vi "1.3.14-ReadWrite.vi"(0 "Read FIFO":refnum<k21>="2.3.2-Lidar Read", 1 "baud rate (9600) 2":u32=9600, 2 "data bits (8) 2":i32=8 min=5 max=8 step=1, 3 "stop bits (10: 1 bit) 2":u16(ring)=10 items=["1.0"=10, "1.5"=15, "2.0"=20], 5 "Write FIFO":refnum<k21>="2.3.1-Lidar Write", 7 "Rx FPGA I/O":refnum<k21>="Rx", 9 "Tx FPGA I/O":refnum<k21>="Tx", 11 "stop bits (10: 1 bit)":u16(ring)=10 items=["1.0"=10, "1.5"=15, "2.0"=20], 12 "Invert Polarity?":bool, 13 "parity (0:none)":enum16{"None", "Odd", "Even", "Mark", "Space"}(ring), 14 "Invert Polarity? 2":bool) -> (4 "Read: Transmission Error":bool, 6 "Read: Transmission Error 2":bool)   [LabVIEW 2010]
uses:
  <vilib>/eio/EIONode/EIONode.xnode
  <vilib>/rvi/eio/nirviEIOImplementation/nirviEIOImplementation.xnode
  <vilib>/rvi/eio/common/nirviEmuClasses.ctl
  <vilib>/rvi/DataTransferAndStorage/Container/XNode/niFpgaContainer.xnode
  <vilib>/rvi/DataTransferAndStorage/Container/Common/niFpgaTransferTypeControl.ctl
  <vilib>/rvi/FIFO/Fifo_Types/niFpgaFifoControlLogicControl.ctl
  <vilib>/rvi/DataTransferAndStorage/Container/Common/niFpgaContainerMethod.ctl
  <vilib>/rvi/DataTransferAndStorage/Container/Common/niFpgaContainerMetaDataKey.ctl
  <vilib>/rvi/DataTransferAndStorage/FIFO/niFpgaPeerToPeerStreamState.ctl
  1.0-Hindbrain Global.vi
  <vilib>/rvi/eio/common/nirviEmuTemplateMethod_noerrors.vi
  <vilib>/rvi/DataTransferAndStorage/Container/Common/niFpgaContainerExecOnDevCompGetState.vi
  <vilib>/rvi/FIFO/Fifo_Resource/nirvififoEmulationSetSize.vi
  <vilib>/rvi/DataTransferAndStorage/Container/Common/niFpgaContainerGetUniqueNameForEmu.vi
  <vilib>/rvi/interface/RandomDataEmulation/nirviRandomDataFPGAFIFO.vi
  <vilib>/rvi/interface/RandomDataEmulation/niFpgaRandomDataHandleErrors.vi
  <vilib>/rvi/eio/common/nirviEmuReportErrorAndStop.vi
panel:
  in  "parity (0:none) 2":enum16{"None", "Odd", "Even", "Mark", "Space"}(ring)
  in  "data bits (8)":i32=8 min=5 max=8 step=1
  in  "baud rate (9600)":u32=9600
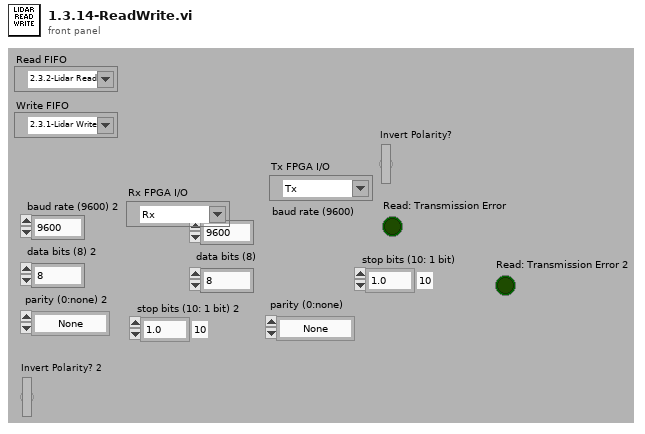
[diagram p1: front panel]
types:
  T1 = typedef "nirviEmuClasses.ctl" = enum16{"IO Read", "IO Write", "Method", "Property Read", "Property Write"}
  T2 = typedef "niFpgaFifoControlLogicControl.ctl" = enum16{"Slice Fabric", "Target Optimal", "Built-in"}
  T3 = typedef "niFpgaContainerMethod.ctl" = enum16{"<none>", "write", "read", "clear", "getNumberOfElementsToWrite", "getNumberOfElementsToRead", "enable", "disable", "flushAndDisable", "getStreamState", "readA", "readB", "dramWrite", "dramWriteWithByteEnables", "dramRequestData", "dramRetrieveData"}
  T4 = typedef "niFpgaTransferTypeControl.ctl" = enum16{"Target-Scoped", "Host to Target - DMA", "Target to Host - DMA", "Peer to Peer Reader", "Peer to Peer Writer", "Bidirectional"}
  T5 = typedef "niFpgaPeerToPeerStreamState.ctl" = enum16{"Unlinked", "Disabled", "Enabled", "Flushing"}
  T6 = typedef "niFpgaContainerMetaDataKey.ctl" = enum16{"FPGA FIFO", "FPGA Memory", "FPGA Register"}
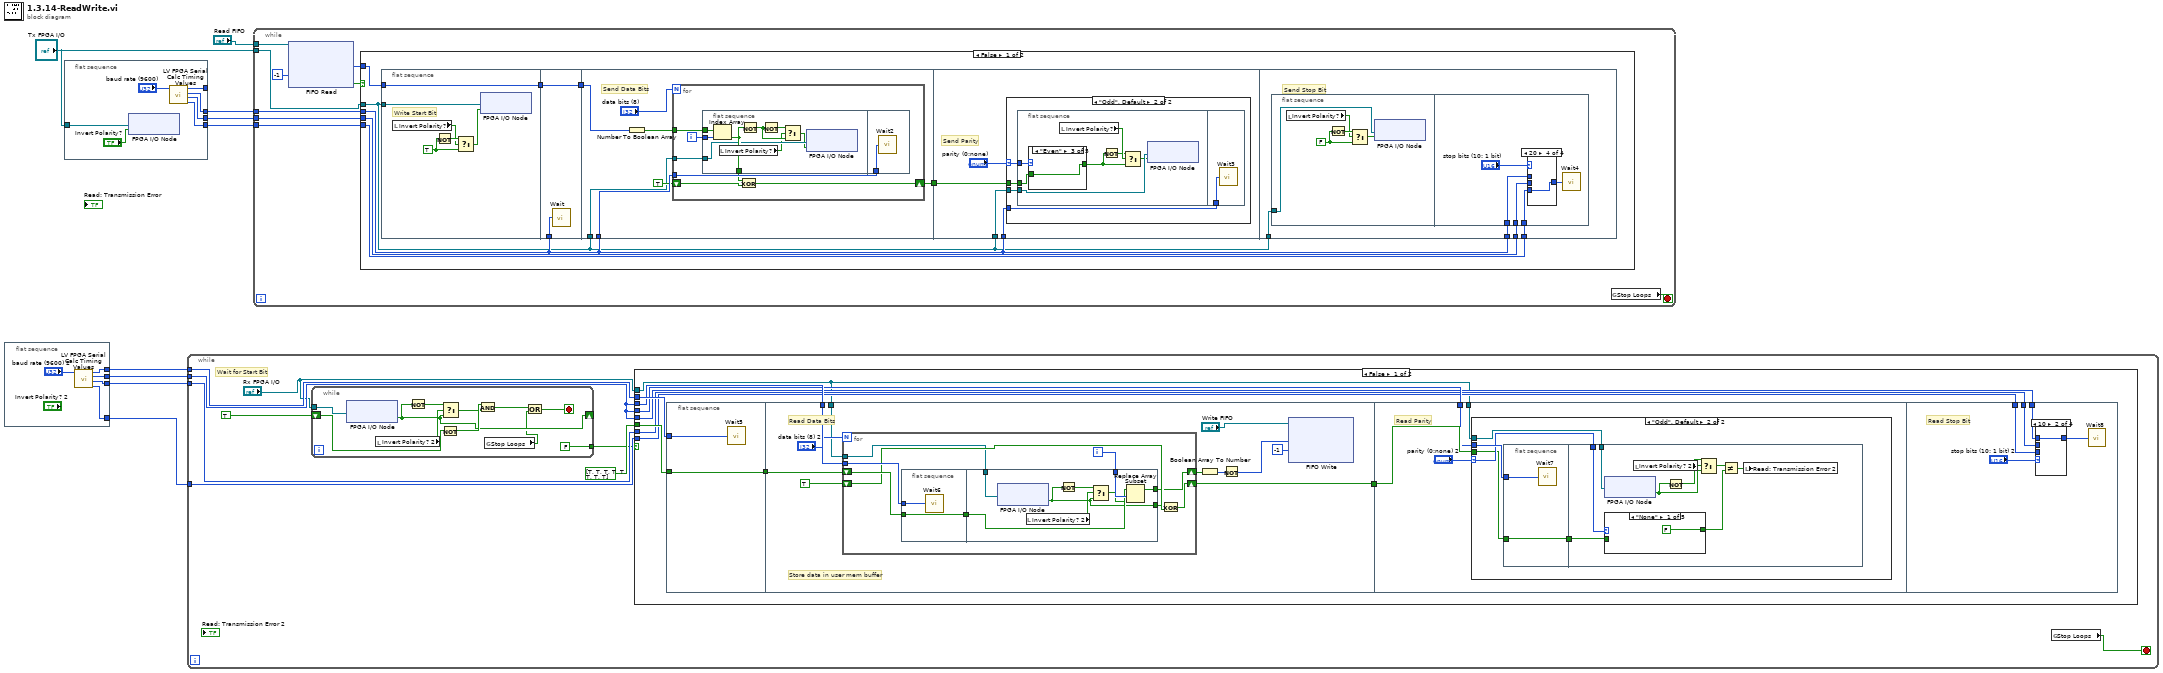
[diagram p0: block diagram]
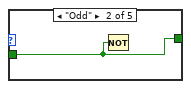
[diagram p3: hidden frame]
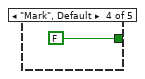
[diagram p5: hidden frame]
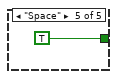
[diagram p6: hidden frame]
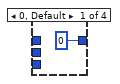
[diagram p7: hidden frame]
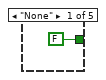
[diagram p12: hidden frame]
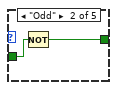
[diagram p13: hidden frame]
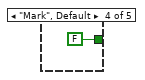
[diagram p14: hidden frame]
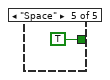
[diagram p15: hidden frame]
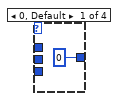
[diagram p16: hidden frame]
diagram:
  n1 = flat-sequence {
    tunnel: [w10] -> w3
    tunnel: [w13] -> w2
    tunnel: [w12] -> w4
    tunnel: [w11] -> w5
    frame #0 {
      n2 = call "LV FPGA Serial Calc Timing Values.vi"("baud rate (1000000)"="baud rate (9600) 2") -> ("Two Bit"=w11:u32, "One and Half Bit"=w12:u32, "One Bit"=w10:u32, "Half Bit"=w13:u32)  [unwired: 1 in, 2 out]
    }
  }
  n3 = flat-sequence {
    tunnel: [w17] -> w9
    tunnel: [w20] -> _
    tunnel: [w19] -> w8
    tunnel: [w18] -> w7
    tunnel: "Tx FPGA I/O" -> [w16]
    frame #0 {
      n4 = xnode "FPGA I/O Node"("I/O Item"="Invert Polarity?", "FPGA I/O In"=w16) -> ()  [unwired: 1 out]
      n5 = call "LV FPGA Serial Calc Timing Values.vi"("baud rate (1000000)"="baud rate (9600)") -> ("Two Bit"=w18:u32, "One and Half Bit"=w19:u32, "One Bit"=w17:u32, "Half Bit"=w20:u32)  [unwired: 1 in, 2 out]
    }
  }
  n6 = while {
    tunnel: w5 -> [w40]
    tunnel: w4 -> [w39]
    tunnel: w3 -> [w38]
    tunnel: w2 -> [w37]
    stop <- w34 stop-if-true
    # "Wait for Start Bit"
    n7 = while {
      tunnel: [FALSE] -> w36
      shift-right: [w43] -> _
      shift-left: TRUE -> [w51]
      tunnel: "Rx FPGA I/O" -> [w47]
      stop <- w48 stop-if-true
      n8 = xnode "FPGA I/O Node"("FPGA I/O In"=w47) -> ("I/O Item"=w43:bool)  [unwired: 1 out]
      n9 = local read "Invert Polarity? 2"() -> (w45:bool)
      n10 = Not(x=w43) -> (.not. x?=w46:bool)
      n11 = Not(x=w51) -> (.not. x?=w50:bool)
      n12 = Select(t=w46, s=w45, f=w43) -> (s? t:f=w44:bool)
      n13 = And(x=w50, y=w44) -> (x .and. y?=w49:bool)
      n14 = global read "1.0-Hindbrain Global.vi" "Stop Loops"() -> (w42:bool)
      n15 = Or(x=w49, y=w42) -> (x .or. y?=w48:bool)
    }
    n16 = case shown="False" w36 {
      tunnel: bool[] [TRUE, TRUE, TRUE, TRUE, TRUE, TRUE, TRUE, TRUE] -> [w80 _]
      tunnel: w37 -> [w79 _]
      tunnel: w38 -> [w78 _]
      tunnel: w38 -> [w77 _]
      tunnel: w38 -> [w76 _]
      tunnel: w39 -> [w75 _]
      tunnel: w40 -> [w74 _]
      tunnel: "Rx FPGA I/O" -> [w72 _]
      frame False {
        n17 = flat-sequence {
          tunnel: [w83] -> w81
          tunnel: w80 -> [w83]
          tunnel: w79 -> [w82]
          tunnel: w81 -> [w94]
          tunnel: w78 -> [w93]
          tunnel: [w89] -> w73
          tunnel: w72 -> [w87]
          tunnel: w77 -> [w451]
          tunnel: w73 -> [w453]
          tunnel: w72 -> [w450]
          tunnel: w76 -> [w497]
          tunnel: w75 -> [w496]
          tunnel: w74 -> [w495]
          frame #0 {
            n18 = call "Wait5"("Count(Ticks)"=w82) -> ()  [unwired: 1 out]
          }
          frame #1 {
            # "Store data in user mem buffer"
            # "Read Data Bits"
            n19 = for {
              N: "data bits (8) 2" -> [_]
              shift-right: [w414] -> w92
              shift-left: w94 -> [w420]
              tunnel: w93 -> [w418]
              shift-right: [w417] -> w89
              shift-left: TRUE -> [w416]
              tunnel: w87 -> [w412]
              i -> [w413]
              n20 = flat-sequence {
                tunnel: w420 -> [w422]
                tunnel: [w422] -> w419
                tunnel: w418 -> [w421]
                tunnel: w413 -> [w430]
                tunnel: w419 -> [w429]
                tunnel: [w428] -> w414
                tunnel: [w423] -> w415
                tunnel: w412 -> [w427]
                frame #0 {
                  n21 = call "Wait6"("Count(Ticks)"=w421) -> ()  [unwired: 1 out]
                }
                frame #1 {
                  n22 = xnode "FPGA I/O Node"("FPGA I/O In"=w427) -> ("I/O Item"=w423:bool)  [unwired: 1 out]
                  n23 = local read "Invert Polarity? 2"() -> (w426:bool)
                  n24 = Not(x=w423) -> (.not. x?=w425:bool)
                  n25 = Select(t=w425, s=w426, f=w423) -> (s? t:f=w424:bool)
                  n26 = Replace Array Subset(array=w429, new element=w424, index=w430) -> (w428:bool[])
                }
              }
              n27 = Exclusive Or(1:w416, 2:w415) -> (0:w417:bool)
            }
            n28 = Boolean Array To Number(Boolean array=w92) -> (number=w91:u8)
            n29 = Not(x=w91) -> (.not. x?=w86:u8)
            n30 = xnode ("FIFO Write")("Element"=w86, "Timeout"=-1, "FIFO In"="Write FIFO") -> ()  [unwired: 2 out]
          }
          frame #2 {
            # "Read Parity"
            n31 = case shown="\"Odd\", Default" "parity (0:none) 2" {
              selector: "parity (0:none) 2" -> [_ w457]
              tunnel: w453 -> [_ w455]
              tunnel: w451 -> [_ w458]
              tunnel: w450 -> [_ w454]
              frame "None" {
              }
              frame "Odd", Default {
                n32 = flat-sequence {
                  tunnel: w458 -> [w460]
                  tunnel: [w459] -> w456
                  tunnel: w455 -> [w459]
                  tunnel: w457 -> [w469]
                  tunnel: w456 -> [w467]
                  tunnel: w454 -> [w465]
                  frame #0 {
                    n33 = call "Wait7"("Count(Ticks)"=w460) -> ()  [unwired: 1 out]
                  }
                  frame #1 {
                    n34 = xnode "FPGA I/O Node"("FPGA I/O In"=w465) -> ("I/O Item"=w462:bool)  [unwired: 1 out]
                    n35 = case shown="\"None\"" w469 {
                      tunnel: w467 -> [_ w490 w491 _ _]
                      tunnel: [FALSE ("y") w490 w491 FALSE ("y") TRUE ("y")] -> w468
                      frame "None" {
                      }
                      frame "Odd" {
                        n36 = Not(x=w490) -> ()  [unwired: 1 out]
                      }
                      frame "Even" {
                      }
                      frame "Mark", Default {
                      }
                      frame "Space" {
                      }
                    }
                    n37 = local read "Invert Polarity? 2"() -> (w463:bool)
                    n38 = Not(x=w462) -> (.not. x?=w464:bool)
                    n39 = Select(t=w464, s=w463, f=w462) -> (s? t:f=w461:bool)
                    n40 = Not Equal?(x=w461, y=w468) -> (x != y?=w466:bool)
                    n41 = local write "Read: Transmission Error 2"(w466) -> ()
                  }
                }
              }
            }
          }
          frame #3 {
            # "Read Stop Bit"
            n42 = case shown="10" "stop bits (10: 1 bit) 2" {
              tunnel: w497 -> [_ w500 _ _]
              tunnel: w496 -> [_ _ w501 _]
              tunnel: w495 -> [_ _ _ w502]
              tunnel: [u32 0 ("One Bit") w500 w501 w502] -> w494
              frame 0, Default {
              }
              frame 10 {
              }
              frame 15 {
              }
              frame 20 {
              }
            }
            n43 = call "Wait8"("Count(Ticks)"=w494) -> ()  [unwired: 1 out]
          }
        }
      }
      frame True {
      }
    }
    n44 = global read "1.0-Hindbrain Global.vi" "Stop Loops"() -> (w34:bool)
  }
  n45 = while {
    tunnel: w7 -> [w511]
    tunnel: w8 -> [w510]
    tunnel: w9 -> [w509]
    tunnel: "Tx FPGA I/O" -> [w508]
    tunnel: "Read FIFO" -> [w503]
    stop <- w504 stop-if-true
    n46 = xnode ("FIFO Read")("Timeout"=-1, "FIFO In"=w503) -> ("Element"=w507:u8, "Timed Out?"=w505:bool)  [unwired: 1 out]
    n47 = case shown="False" w505 {
      tunnel: w511 -> [w833 _]
      tunnel: w510 -> [w832 _]
      tunnel: w509 -> [w831 _]
      tunnel: w508 -> [w830 _]
      tunnel: w507 -> [w829 _]
      frame False {
        n48 = flat-sequence {
          tunnel: w830 -> [w842]
          tunnel: w829 -> [w837]
          tunnel: [w837] -> w836
          tunnel: w831 -> [w855]
          tunnel: [w854] -> w835
          tunnel: w836 -> [w854]
          tunnel: w831 -> [w862]
          tunnel: [w860] -> w834
          tunnel: w830 -> [w858]
          tunnel: w835 -> [w857]
          tunnel: w831 -> [w892]
          tunnel: w834 -> [w893]
          tunnel: w830 -> [w891]
          tunnel: w831 -> [w926]
          tunnel: w832 -> [w925]
          tunnel: w833 -> [w924]
          tunnel: w830 -> [w923]
          frame #0 {
            w840 = TRUE
            # "Write Start Bit"
            n49 = local read "Invert Polarity?"() -> (w839:bool)
            n50 = Not(x=w840) -> (.not. x?=w841:bool)
            n51 = Select(t=w841, s=w839, f=w840) -> (s? t:f=w838:bool)
            n52 = xnode "FPGA I/O Node"("I/O Item"=w838, "FPGA I/O In"=w842) -> ()  [unwired: 1 out]
          }
          frame #1 {
            n53 = call "Wait"("Count(Ticks)"=w855) -> ()  [unwired: 1 out]
          }
          frame #2 {
            # "Send Data Bits"
            n54 = Number To Boolean Array(number=w857) -> (Boolean array=w859:bool[])
            n55 = for {
              N: "data bits (8)" -> [_]
              tunnel: w862 -> [w866]
              shift-right: [w869] -> w860
              shift-left: TRUE -> [w868]
              tunnel: w859 -> [w865]
              tunnel: w858 -> [w863]
              i -> [w867]
              n56 = flat-sequence {
                tunnel: w867 -> [w877]
                tunnel: w865 -> [w876]
                tunnel: [w875] -> w864
                tunnel: w863 -> [w874]
                tunnel: w866 -> [w889]
                frame #0 {
                  n57 = Index Array(array=w876, index=w877) -> (element=w875:bool)
                  n58 = local read "Invert Polarity?"() -> (w871:bool)
                  n59 = Not(x=w875) -> (.not. x?=w872:bool)
                  n60 = Not(x=w872) -> (.not. x?=w873:bool)
                  n61 = Select(t=w873, s=w871, f=w872) -> (s? t:f=w870:bool)
                  n62 = xnode "FPGA I/O Node"("I/O Item"=w870, "FPGA I/O In"=w874) -> ()  [unwired: 1 out]
                }
                frame #1 {
                  n63 = call "Wait2"("Count(Ticks)"=w889) -> ()  [unwired: 1 out]
                }
              }
              n64 = Exclusive Or(1:w868, 2:w864) -> (0:w869:bool)
            }
          }
          frame #3 {
            # "Send Parity"
            n65 = case shown="\"Odd\", Default" "parity (0:none)" {
              selector: "parity (0:none)" -> [_ w897]
              tunnel: w893 -> [_ w896]
              tunnel: w892 -> [_ w895]
              tunnel: w891 -> [_ w894]
              frame "None" {
              }
              frame "Odd", Default {
                n66 = flat-sequence {
                  tunnel: w896 -> [w903]
                  tunnel: w897 -> [w904]
                  tunnel: w894 -> [w902]
                  tunnel: w895 -> [w922]
                  frame #0 {
                    n67 = case shown="\"Even\"" w904 {
                      tunnel: w903 -> [_ w918 w919 _ _]
                      tunnel: [FALSE ("y") w917 w919 FALSE ("y") TRUE ("y")] -> w899
                      frame "None" {
                      }
                      frame "Odd" {
                        n68 = Not(x=w918) -> (.not. x?=w917:bool)
                      }
                      frame "Even" {
                      }
                      frame "Mark", Default {
                      }
                      frame "Space" {
                      }
                    }
                    n69 = local read "Invert Polarity?"() -> (w901:bool)
                    n70 = Not(x=w899) -> (.not. x?=w900:bool)
                    n71 = Select(t=w900, s=w901, f=w899) -> (s? t:f=w898:bool)
                    n72 = xnode "FPGA I/O Node"("I/O Item"=w898, "FPGA I/O In"=w902) -> ()  [unwired: 1 out]
                  }
                  frame #1 {
                    n73 = call "Wait3"("Count(Ticks)"=w922) -> ()  [unwired: 1 out]
                  }
                }
              }
            }
          }
          frame #4 {
            # "Send Stop Bit"
            n74 = flat-sequence {
              tunnel: w923 -> [w931]
              tunnel: w926 -> [w947]
              tunnel: w925 -> [w946]
              tunnel: w924 -> [w945]
              frame #0 {
                w929 = FALSE
                n75 = local read "Invert Polarity?"() -> (w928:bool)
                n76 = Not(x=w929) -> (.not. x?=w930:bool)
                n77 = Select(t=w930, s=w928, f=w929) -> (s? t:f=w927:bool)
                n78 = xnode "FPGA I/O Node"("I/O Item"=w927, "FPGA I/O In"=w931) -> ()  [unwired: 1 out]
              }
              frame #1 {
                n79 = case shown="20" "stop bits (10: 1 bit)" {
                  tunnel: w947 -> [_ w949 _ _]
                  tunnel: w946 -> [_ _ w950 _]
                  tunnel: w945 -> [_ _ _ w951]
                  tunnel: [u32 0 ("One Bit") w949 w950 w951] -> w944
                  frame 0, Default {
                  }
                  frame 10 {
                  }
                  frame 15 {
                  }
                  frame 20 {
                  }
                }
                n80 = call "Wait4"("Count(Ticks)"=w944) -> ()  [unwired: 1 out]
              }
            }
          }
        }
      }
      frame True {
      }
    }
    n81 = global read "1.0-Hindbrain Global.vi" "Stop Loops"() -> (w504:bool)
  }
